vi "Log_File_Init.vi"(0 "Data File Directory":path=path "c:/data", 1 "extension":string="tmp", 5 "Test Type":string="FIRST HOUR DELIVERY", 7 "Device ID":string="GE HEWH 1", 9 "Run":i32=1, 11 "error in (no error)":errorcluster, 12 "Runtime Version":string="GE HEWH 1", 13 "Computer Name":string="0-President") -> (6 "FileName":path, 15 "error out":errorcluster)   [LabVIEW 2009]
uses:
  <vilib>/Utility/file.llb/Write To Spreadsheet File (string).vi
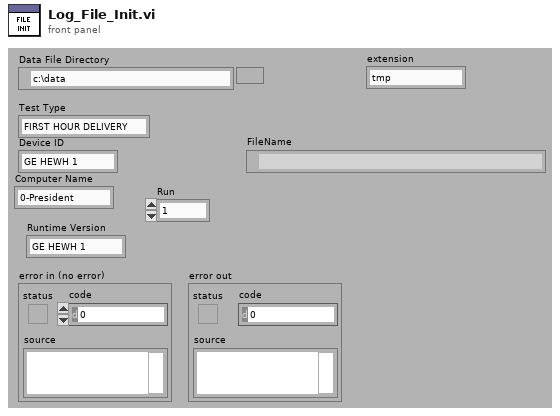
[diagram p1: front panel]
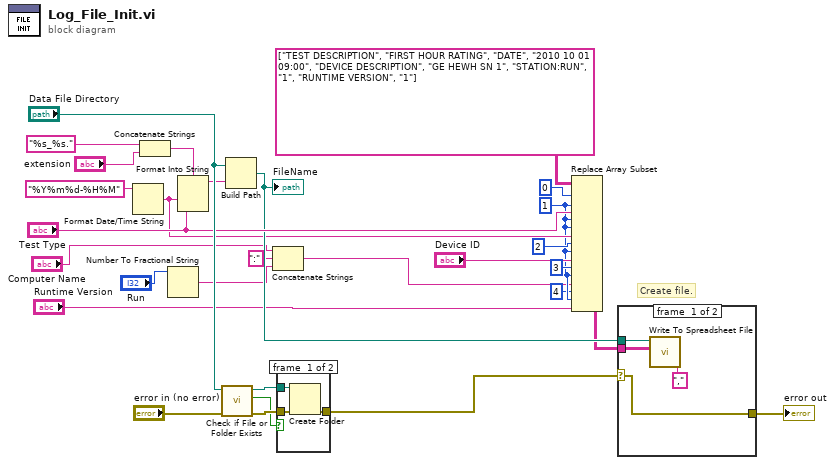
[diagram p0: block diagram]
diagram:
  w7 = 1 ("disabled index (col)")
  # "Create file."
  n1 = Format Date/Time String(time format string (%c)="%Y%m%d-%H%M") -> (date/time string=w8:string)  [unwired: 2 out]
  n2 = Concatenate Strings("%s_%s." ("format string"), "extension") -> (w28:string)
  n3 = Number To Fractional String(number="Run") -> (F-format string=w2:string)  [unwired: 3 in]
  n4 = Format Into String(format string=w28, w8, "Test Type") -> (resulting string=w25:string)  [unwired: 2 in, 1 out]
  n5 = call <vilib>:"Check if File or Folder Exists.vi"("error in (no error)"="error in (no error)", "path"="Data File Directory") -> ("error out"=w23:errorcluster, "file or folder exists?"=w11:bool, "dup path"=w22:path)  [unwired: 7 out]
  n6 = Build Path(base path="Data File Directory", name or relative path=w25) -> (appended path=w13:path)
  "FileName" <- w13
  n7 = Concatenate Strings("Computer Name", ":" ("string"), w2) -> (w1:string)
  n8 = case shown="False" w11 {
    tunnel: w22 -> [w30 _]
    tunnel: w23 -> [w32 w33]
    tunnel: [w31 w33] -> w10
    frame #0 {
      n9 = Create Folder(path (use dialog)=w30, error in=w32) -> (error out=w31:errorcluster)  [unwired: 3 out]
    }
    frame #1 {
    }
  }
  n10 = Replace Array Subset(array=string[][] [["TEST DESCRIPTION", "FIRST HOUR RATING"], ["DATE", "2010 10 01 09:00"], ["DEVICE DESCRIPTION", "GE HEWH SN 1"], ["STATION:RUN", "1"], ["RUNTIME VERSION", "1"]], new element #1="Test Type", index (row) #1=0 ("index (row)"), index (col) #1=w7, new element #2=w8, index (row) #2=w7, index (col) #2=w7, new element #3="Device ID", index (row) #3=2 ("disabled index (row)"), index (col) #3=w7, new element #4=w1, index (row) #4=3 ("disabled index (row)"), index (col) #4=w7, new element #5="Runtime Version", index (row) #5=4 ("disabled index (row)"), index (col) #5=w7) -> (w12:string[][])
  n11 = case shown="No Error" w10 {
    selector: w10 -> [w34 w38]
    tunnel: w13 -> [w37 _]
    tunnel: w12 -> [w36 _]
    tunnel: [w34 w38] -> w9
    frame #0 {
      n12 = call-poly <vilib>:"Write To Spreadsheet File.vi"("delimiter (\\t)"="," ("delimiter (\\t)"), "2D data"=w36, "file path (dialog if empty)"=w37) -> ()  [unwired: 5 in, 1 out]
    }
    frame #1 {
    }
  }
  "error out" <- w9
